vi "SV TDMS Read Scalar (1 Ch).vi"(0 "tdms file":refnum<k34>, 1 "offset (0)":i64, 2 "count (-1: all)":i64=-1, 5 "group name in":string, 7 "channel name in":string, 11 "error in":errorcluster) -> (3 "scale labels":T1, 4 "tdms file out":refnum<k34>, 6 "group name out":string, 8 "channel name out":string, 10 "values":dbl[](array[numeric]), 13 "scalar function info":T2={"scalar function type"=10, "scalar function subtype"=19, " x-dimension"=0} {"scalar function type" items=["Speed"=3, "Ratio"=6, "Count"=7, "-"=9, "Level"=10, "-"=19, "None"=98]; "scalar function subtype" items=["Value"=19, "DC"=11, "AC"=12, "RMS^2"=13, "RMS"=14, "Peak"=15, "Peak to peak"=16, "-"=20, "Phase"=33, "-"=90, "None"=98, "Unknown"=99]; "x-dimension" items=["Time (s)"=0, "Frequency-CB (Hz)"=1, "Frequency-CPB (Hz)"=1248, "Frequency-Arbitrary (Hz)"=2357, "Quefrency (s)"=2, "Revolutions (rev)"=3, "Order"=4, "Speed (RPM)"=11, "Speed (rad/s)"=21, "Critical Band"=31, "Critical Band Rate (Bark)"=32, "None"=98, "Index"=65535]}, 14 "end of file":bool, 15 "error out":errorcluster)   [LabVIEW 2017]
doc: "Reads the specified .tdms file and returns data in a format specific to the polymorphic instance selected."
uses:
  <vilib>/addons/_NISVFA/_Shared subVIs/Controls/NI Scalar Function Info.ctl
  <vilib>/addons/_NISVFA/_Shared subVIs/Controls/svc_X-Axis Units.ctl
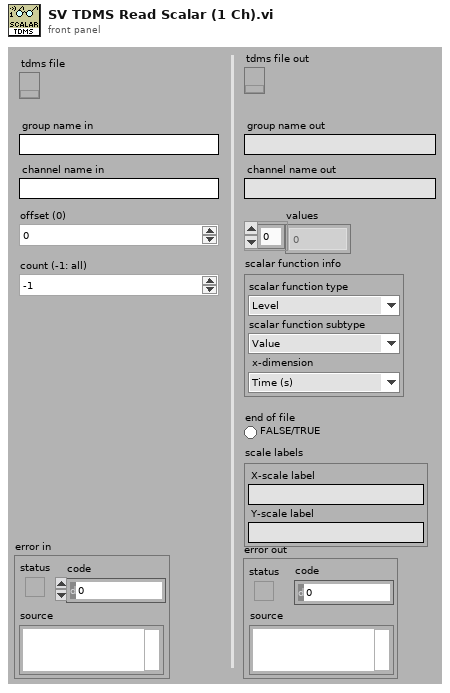
[diagram p1: front panel]
types:
  T1 = cluster{"X-scale label":string, "Y-scale label":string}
  T2 = typedef "NI Scalar Function Info.ctl" = cluster{"scalar function type":u16, "scalar function subtype":u16, " x-dimension":T3}
  T3 = typedef "svc_X-Axis Units.ctl" = u16
  T4 = typedef "NI Function Info.ctl" = cluster{"function type":T5, "function subtype":T6, "X-dimension":T3}
  T5 = typedef "NI Function Type.ctl" = u16
  T6 = typedef "NI Function SubType.ctl" = u16
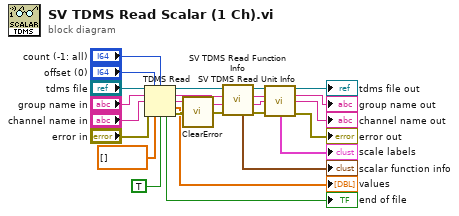
[diagram p0: block diagram]
diagram:
  n1 = TDMS Read(0:"tdms file", 1:"offset (0)", 2:"count (-1: all)", 5:"group name in", 7:"channel name in", 11:"error in", 12:dbl[] [], 13:TRUE ("return channels in file order? (F)")) -> (4:w14:refnum<k34>, 6:w13:string, 8:w12:string, 10:→"values":dbl[], 14:→"end of file":bool, 15:w18:errorcluster)
  n2 = call <vilib>:"ClearError.vi"("error in (no error)"=w18) -> ("error out"=w8:errorcluster)
  n3 = call <vilib>:"SV TDMS Read Function Info.vi"("error in (no error)"=w8, "channel name"=w12, "group name"=w13, "tdms file in"=w14) -> ("error out"=w7:errorcluster, "channel name out"=w10:string, "group name out"=w11:string, "tdms file out"=w9:refnum<k34>, "function info"=→"scalar function info":T4)  [unwired: 2 in, 1 out]
  n4 = call <vilib>:"SV TDMS Read Unit Info.vi"("tdms file"=w9, "group name"=w11, "channel name"=w10, "error in (no error)"=w7) -> ("tdms file out"=→"tdms file out":refnum<k34>, "group name out"=→"group name out":string, "channel name out"=→"channel name out":string, "scale labels"=→"scale labels":T1, "error out"=→"error out":errorcluster)  [unwired: 6 in, 1 out]
